vi "SolutionBuilder.vi"(11 "Path":path) -> (3 "status":bool=TRUE)   [LabVIEW 2019]
uses:
  SolutionBuilder/SolutionBuilder.lvclass
  SolutionBuilder/SolutionBuilder.lvlib
panel:
  out "source":string="Empty path input."
  out "code":i32=7
  out "Results":i32(listbox)=-1
  in  "Preview?":bool
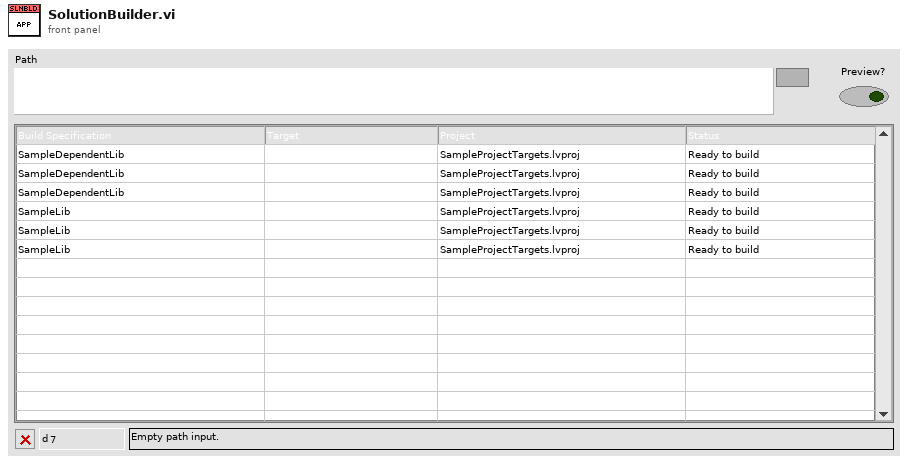
[diagram p1: front panel]
types:
  T1 = typedef "SolutionBuilder.lvlib/Events.ctl" = cluster{"UpdateList":T2, "ItemBuilt":T3, "Stop":refnum<user-event>}
  T2 = typedef "SolutionBuilder.lvlib/EventUpdateList.ctl" = refnum<user-event>
  T3 = typedef "SolutionBuilder.lvlib/EventItemBuilt.ctl" = refnum<user-event>
  T4 = typedef "SolutionBuilder.lvlib/BuildManager.lvclass/GeneratedFile.ctl" = cluster{"Project path":path, "Build spec name":string, "Path":path}
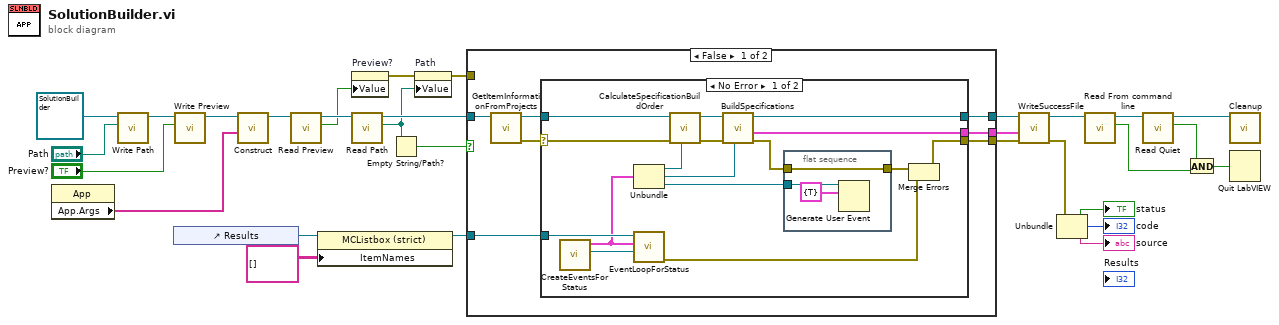
[diagram p0: block diagram]
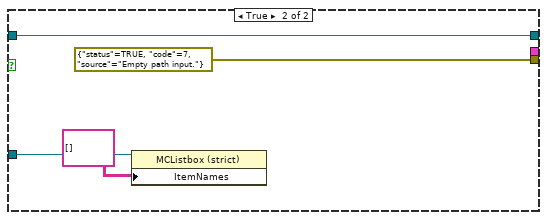
[diagram p3: hidden frame]
diagram:
  n1 = property class="App"() -> ("App.Args"=w1:string[])  [unwired: 2 in, 2 out]
  n2 = call-dynamic "Write Path.vi"("Path"="Path", "SolutionBuilder in"=refnum<class "SolutionBuilder.lvclass"> refnum) -> ("SolutionBuilder out"=w30:refnum<class "SolutionBuilder.lvclass">)  [unwired: 9 in]
  n3 = control-ref of="Results"() -> (w10:refnum<vi>)
  n4 = call-dynamic "Write Preview.vi"("Preview?"="Preview?", "SolutionBuilder in"=w30) -> ("SolutionBuilder out"=w28:refnum<class "SolutionBuilder.lvclass">)  [unwired: 9 in]
  n5 = call-dynamic "Construct.vi"("App.Args"=w1, "SolutionBuilder in"=w28) -> ("SolutionBuilder out"=w16:refnum<class "SolutionBuilder.lvclass">)  [unwired: 8 in, 1 out]
  n6 = call-dynamic "Read Preview.vi"("SolutionBuilder in"=w16) -> ("Preview?"=w11:bool, "SolutionBuilder out"=w15:refnum<class "SolutionBuilder.lvclass">)  [unwired: 9 in]
  n7 = property class="MCListbox (strict)"(reference=w10, "ItemNames"=string[][] [] ("Item Names")) -> (reference out=w9:refnum<vi>)  [unwired: 1 in, 1 out]
  n8 = property on="Preview?" class="Bool (strict)"("Value"=w11) -> (error out=w12:errorcluster)  [unwired: 2 in, 1 out]
  n9 = call-dynamic "Read Path.vi"("SolutionBuilder in"=w15) -> ("Path"=w14:path, "SolutionBuilder out"=w23:refnum<class "SolutionBuilder.lvclass">)  [unwired: 9 in]
  n10 = Empty String/Path?(string/path=w14) -> (empty?=w24:bool)
  n11 = property on="Path" class="Path"(error in=w12, "Value"=w14) -> (error out=w13:errorcluster)  [unwired: 1 in, 1 out]
  n12 = case shown="False" w24 {
    tunnel: [w37 errorcluster {"status"=TRUE, "code"=7, "source"="Empty path input."} ("t")] -> w4
    tunnel: w9 -> [w36 w60]
    tunnel: w23 -> [w32 w59]
    tunnel: [w35 w59] -> w6
    tunnel: w13 -> [_ _]
    tunnel: [w31 _] -> w3
    frame False {
      n13 = call-dynamic "GetItemInformationFromProjects.vi"("SolutionBuilder in"=w32) -> ("error out"=w33:errorcluster, "SolutionBuilder out"=w34:refnum<class "SolutionBuilder.lvclass">)  [unwired: 9 in]
      n14 = case shown="No Error" w33 {
        selector: w33 -> [w43 w57]
        tunnel: w36 -> [w47 _]
        tunnel: w34 -> [w46 w58]
        tunnel: [w45 w58] -> w35
        tunnel: [w44 w57] -> w37
        tunnel: [w38 _] -> w31
        frame No Error {
          n15 = call "CreateEventsForStatus.vi"() -> ("Event Registration Refnum"=w39:refnum<event-registration>, "Events"=w40:T1)  [unwired: 10 in]
          n16 = Unbundle(w40) -> ("UpdateList"=w53:T2, "ItemBuilt"=w50:T3, "Stop"=w51:refnum<user-event>)
          n17 = call "EventLoopForStatus.vi"("Event Registration Refnum"=w39, "Events"=w40, "MulticolumnListbox in"=w47) -> ("error out"=w52:errorcluster)  [unwired: 8 in]
          n18 = call-dynamic "CalculateSpecificationBuildOrder.vi"("UpdateList"=w53, "error in (no error)"=w43, "SolutionBuilder in"=w46) -> ("error out"=w49:errorcluster, "SolutionBuilder out"=w48:refnum<class "SolutionBuilder.lvclass">)  [unwired: 7 in]
          n19 = call-dynamic "BuildSpecifications.vi"("ItemBuilt"=w50, "error in (no error)"=w49, "SolutionBuilder in"=w48) -> ("error out"=w41:errorcluster, "Generated files"=w38:T4[], "SolutionBuilder out"=w45:refnum<class "SolutionBuilder.lvclass">)  [unwired: 6 in]
          n20 = flat-sequence {
            tunnel: w51 -> [w55]
            tunnel: [w54] -> w42
            tunnel: w41 -> [w54]
            frame #0 {
              n21 = Generate User Event(user event=w55, event data cluster=cluster{"Stop":bool} {"Stop"=TRUE} ("event data")) -> ()  [unwired: 2 in, 2 out]
            }
          }
          n22 = Merge Errors(w42, w52) -> (w44:errorcluster)
        }
        frame Error {
        }
      }
    }
    frame True {
      n23 = property class="MCListbox (strict)"(reference=w60, "ItemNames"=string[][] [] ("Item Names")) -> ()  [unwired: 1 in, 2 out]
    }
  }
  n24 = call-dynamic "WriteSuccessFile.vi"("error in (no error)"=w4, "Generated files"=w3, "SolutionBuilder in"=w6) -> ("error out"=w2:errorcluster, "SolutionBuilder out"=w5:refnum<class "SolutionBuilder.lvclass">)  [unwired: 7 in]
  n25 = Unbundle(w2) -> ("status"=→"status":bool, "code"=→"code":i32, "source"=→"source":string)
  n26 = call-dynamic "Read From command line.vi"("SolutionBuilder in"=w5) -> ("From command line?"=w17:bool, "SolutionBuilder out"=w19:refnum<class "SolutionBuilder.lvclass">)  [unwired: 9 in]
  n27 = call-dynamic "Read Quiet.vi"("SolutionBuilder in"=w19) -> ("Quiet?"=w18:bool, "SolutionBuilder out"=w25:refnum<class "SolutionBuilder.lvclass">)  [unwired: 9 in]
  n28 = And(x=w18, y=w17) -> (x .and. y?=w7:bool)
  n29 = call-dynamic "Cleanup.vi"("SolutionBuilder in"=w25) -> ()  [unwired: 9 in, 2 out]
  n30 = Quit LabVIEW(quit? (T)=w7) -> ()
